vi "globalSetUp.vi"(8 "error in (no error)":errorcluster, 11 "testcase-CSMArgument in":refnum<class "testcase-issue.lvclass">) -> (0 "error out":errorcluster, 3 "testcase-CSMArgument out":refnum<class "testcase-issue.lvclass">)   [LabVIEW 2017, in "testcase-issue.lvclass"]
uses:
  testcase-issue.lvclass
  <vilib>/addons/_JKI Toolkits/VI Tester/TestCase.llb/TestCase.lvclass
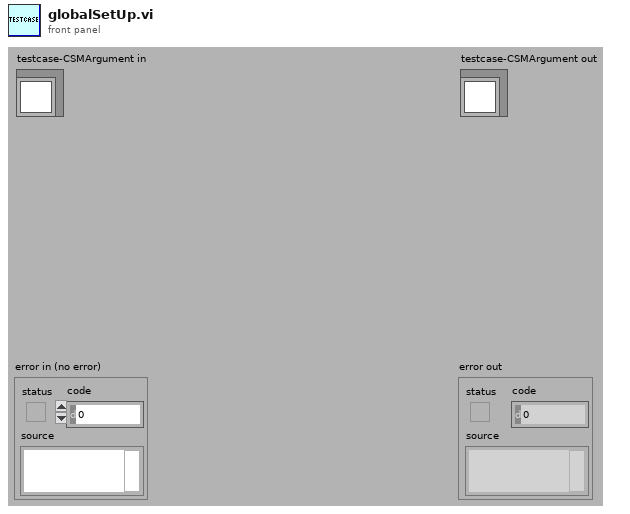
[diagram p1: front panel]
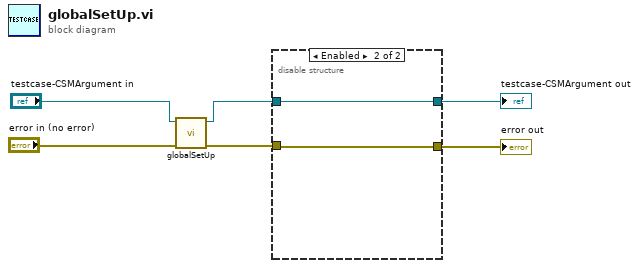
[diagram p0: block diagram]
diagram:
  n1 = call-parent "globalSetUp.vi"("error in (no error)"="error in (no error)", "TestCase in"="testcase-CSMArgument in") -> ("error out"=w3:errorcluster, "TestCase out"=w1:refnum<class "testcase-issue.lvclass">)  [unwired: 8 in]
  n2 = disable-structure shown="Enabled" {
    disable-tunnel: w1 -> [w8 w9]
    disable-tunnel: [w8 w9] -> w6
    disable-tunnel: w3 -> [w7 w10]
    disable-tunnel: [w7 w10] -> w5
    frame Disabled {
    }
    frame Enabled {
    }
  }
  "error out" <- w5
  "testcase-CSMArgument out" <- w6
